vi "8XY7.vi"(11 "Variables and Memory in":T1 {"GFX" format="%02x"}) -> (3 "Variables and Memory out":T1 {"GFX" format="%02x"})   [LabVIEW 2021]
uses:
  Controls/ClusterF.ctl
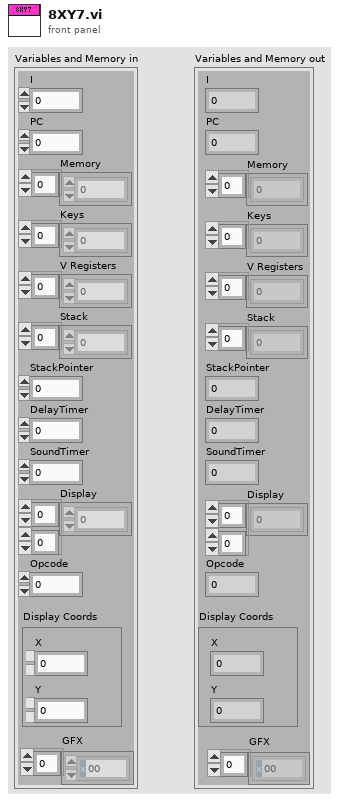
[diagram p1: front panel]
types:
  T1 = typedef "ClusterF.ctl" = cluster{"I":u16, "PC":u16, "Memory":u8[], "Keys":u8[], "V Registers":u8[], "Stack":u16[], "StackPointer":u16, "DelayTimer":u8, "SoundTimer":u8, "Display":u8[][], "Opcode":u16, "Display Coords":cluster{"X":u8, "Y":u8}, "GFX":u8[]}
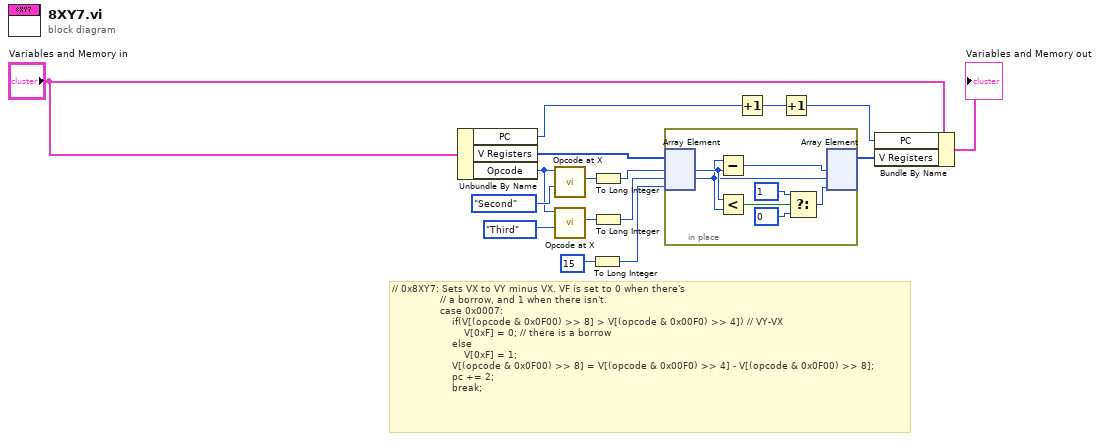
[diagram p0: block diagram]
diagram:
  # "// 0x8XY7: Sets VX to VY minus VX. VF is set to 0 when there's\n                // a borrow, and 1 when there isn't.\n                case 0x0007:\n                    if(V[(opcode & 0x0F00) >> 8] > V[(opcode & 0x00F0) >> 4])\t// VY-VX\n                        V[0xF] = 0; // there is a borrow\n                    else\n                        V[0xF] = 1;\n                    V[(opcode & 0x0F00) >> 8] = V[(opcode & 0x00F0) >> 4] - V[(opcode & 0x0F00) >> 8];\n                    pc += 2;\n                    break;"
  n1 = Unbundle By Name("Variables and Memory in") -> ("PC"=w8:u16, "V Registers"=w6:u8[], "Opcode"=w3:u16)
  n2 = call "Opcode at X.vi"("X Position"=enum16{"First", "Second", "Third", "Fourth"}."Second", "Opcode"=w3) -> ("Opcode at X Position (U8)"=w10:u8)  [unwired: 9 in]
  n3 = call "Opcode at X.vi"("X Position"=enum16{"First", "Second", "Third", "Fourth"}."Third", "Opcode"=w3) -> ("Opcode at X Position (U8)"=w11:u8)  [unwired: 9 in]
  n4 = To Long Integer(number=15) -> (32bit integer=w15:i32)
  n5 = To Long Integer(number=w10) -> (32bit integer=w12:i32)
  n6 = To Long Integer(number=w11) -> (32bit integer=w13:i32)
  n7 = in-place {
    n8 = in-place-array #1(w6, w12, w13, w15) -> (w19:u8, w17:u8)  [unwired: 1 out]
    n9 = Subtract(x=w17, y=w19) -> (x-y=w18:u8)
    n10 = Less?(x=w19, y=w17) -> (x < y?=w23:bool)
    n11 = Select(t=u8 1, s=w23, f=u8 0) -> (s? t:f=w20:u8)
    n12 = in-place-array #1(w18, w17, w20) -> (w16:u8[])  [unwired: 3 out]
  }
  n13 = Increment(x=w8) -> (x+1=w7:u16)
  n14 = Increment(x=w7) -> (x+1=w9:u16)
  n15 = Bundle By Name(cluster="Variables and Memory in", "PC"=w9, "V Registers"=w16) -> (→"Variables and Memory out":T1)
